vi "svx_Orbit and Timebase Segment (N Ch - M Orders).vi"(5 "reset? (F)":bool, 6 "end reach?":bool, 8 "error in (no error)":errorcluster, 9 "indice":cluster{"start":i32, "length":i32}, 11 "order data":dbl[][][](array[numeric])) -> (0 "error out":errorcluster, 3 "order data out":dbl[][][](array[numeric]))   [LabVIEW 2017]
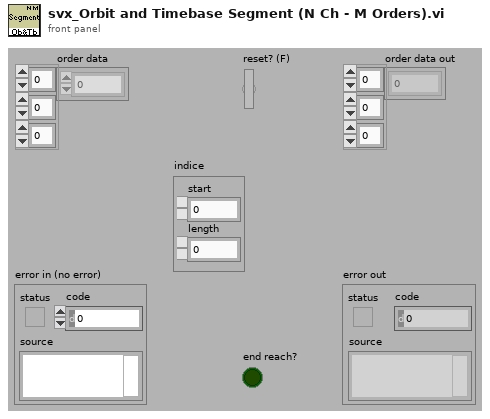
[diagram p1: front panel]
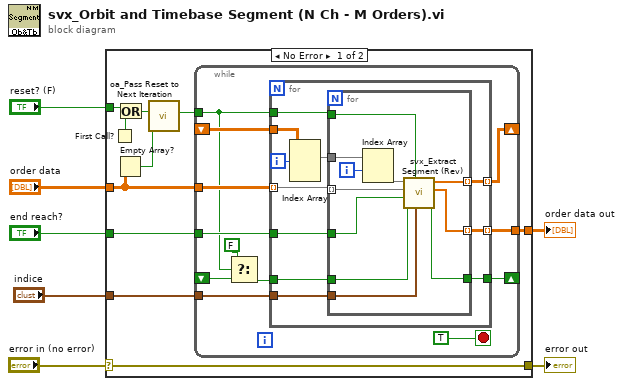
[diagram p0: block diagram]
diagram:
  n1 = case shown="No Error" "error in (no error)" {
    selector: "error in (no error)" -> [w15 w52]
    tunnel: "order data" -> [w14 _]
    tunnel: "reset? (F)" -> [w17 _]
    tunnel: [w15 w52] -> w4
    tunnel: "end reach?" -> [w10 _]
    tunnel: "indice" -> [w9 _]
    tunnel: [w8 _] -> w2
    frame No Error {
      n2 = First Call?() -> (First Call?: T/F=w16:bool)
      n3 = Empty Array?(array=w14) -> (empty?=w12:bool)
      n4 = Or(x=w17, y=w16) -> (x .or. y?=w13:bool)
      n5 = call <vilib>:"oa_Pass Reset to Next Iteration.vi"("trigger"=w12, "reset?(F)"=w13) -> ("reset out"=w11:bool)  [unwired: 9 in]
      n6 = while {
        tunnel: w14 -> [w28]
        shift-right: [w26] -> _
        shift-left: _ -> [w27]
        tunnel: w11 -> [w19]
        shift-right: [w24] -> _
        shift-left: _ -> [w20]
        tunnel: w10 -> [w25]
        tunnel: w9 -> [w23]
        tunnel: [w22] -> w8
        stop <- TRUE stop-if-true
        n7 = Select(t=FALSE, s=w19, f=w20) -> (s? t:f=w21:bool)
        n8 = for {
          tunnel: w28 -> [w40] mode=indexing
          tunnel: w27 -> [w36]
          tunnel: w19 -> [w39]
          tunnel: [w38] -> w24
          tunnel: [w37] -> w26 mode=indexing
          tunnel: w25 -> [w33]
          tunnel: w21 -> [w32]
          tunnel: w23 -> [w31]
          tunnel: [w30] -> w22 mode=indexing
          i -> [w35]
          n9 = Index Array(array=w36, index (dim 0)=w35) -> (element=w34:dbl[][])  [unwired: 2 in]
          n10 = for {
            tunnel: w40 -> [w49] mode=indexing
            tunnel: w34 -> [w51]
            tunnel: w39 -> [w45]
            tunnel: [w42] -> w38
            tunnel: [w48] -> w37 mode=indexing
            tunnel: w33 -> [w44]
            tunnel: w32 -> [w41]
            tunnel: w31 -> [w43]
            tunnel: [w47] -> w30 mode=indexing
            i -> [w50]
            n11 = Index Array(array=w51, index (row)=w50) -> (element=w46:dbl[])  [unwired: 1 in]
            n12 = call <vilib>:"svx_Extract Segment (Rev).vi"("indice"=w43, "reset?"=w45, "old end reached"=w41, "end reached"=w44, "data in"=w49, "old order data"=w46) -> ("end reached out"=w42:bool, "data out"=w47:dbl[], "remaining data"=w48:dbl[])  [unwired: 3 in]
          }
        }
      }
    }
    frame Error {
    }
  }
  "order data out" <- w2
  "error out" <- w4
